vi "BRig_Host_dataRunState__entryDelete__delDataPlot.vi"(7 "input_idx":i32[](array[numeric]), 8 "input_col_dataPlot":u16, 9 "input_row_dataPlot":u16, 11 "input_dataPlot":u16[][](array[numeric])) -> (0 "output_arrTrials":bool, 3 "output_dataPlot":u16[][](array[numeric]), 4 "output_arrTrials_length":i32, 5 "output_idx":i32[](array[numeric]), 6 "output_arrTrials":i32[](array[numeric]))   [LabVIEW 2014]
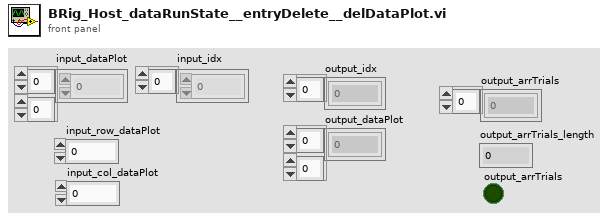
[diagram p1: front panel]
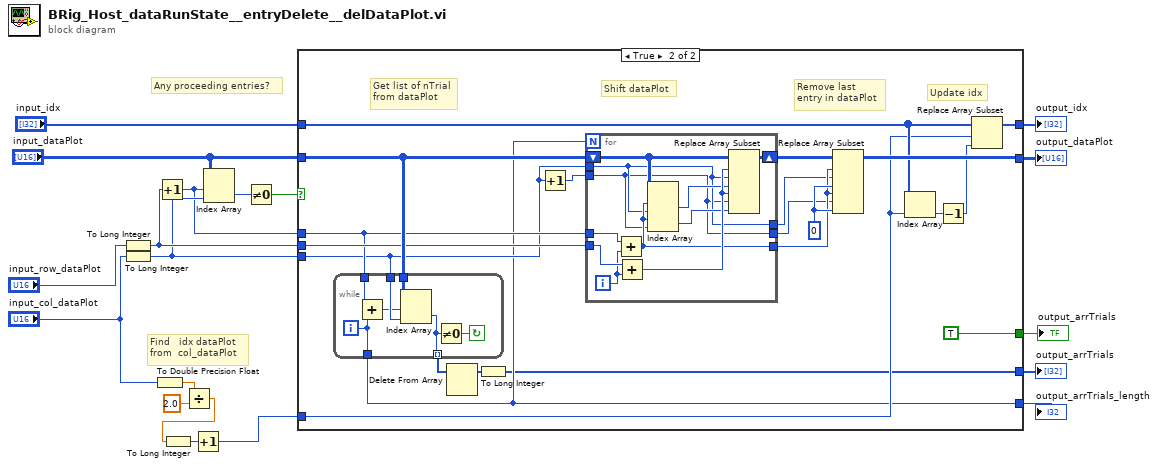
[diagram p0: block diagram]
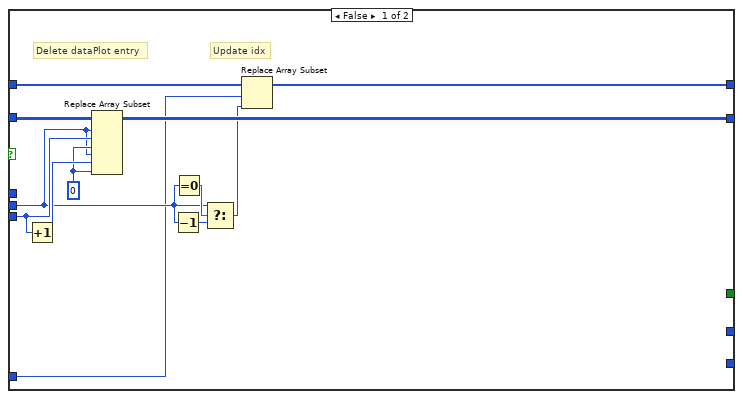
[diagram p2: hidden frame]
diagram:
  # "Find   idx dataPlot\nfrom  col_dataPlot"
  # "Any proceeding entries?"
  n1 = To Long Integer(number="input_row_dataPlot") -> (32bit integer=w14:i32)
  n2 = To Long Integer(number="input_col_dataPlot") -> (32bit integer=w13:i32)
  n3 = To Double Precision Float(number="input_col_dataPlot") -> (double precision float=w11:dbl)
  n4 = Increment(x=w14) -> (x+1=w12:i32)
  n5 = Divide(x=w11, y=2.0) -> (x/y=w9:dbl)
  n6 = To Long Integer(number=w9) -> (32bit integer=w8:i32)
  n7 = Increment(x=w8) -> (x+1=w6:i32)
  n8 = Index Array(array="input_dataPlot", index (row)=w12, index (col)=w13) -> (element=w18:u16)
  n9 = Not Equal To 0?(x=w18) -> (x != 0?=w17:bool)
  n10 = case shown="True" w17 {
    tunnel: "input_dataPlot" -> [w31 w51]
    tunnel: "input_idx" -> [w26 w39]
    tunnel: w14 -> [w22 w50]
    tunnel: w13 -> [w27 w48]
    tunnel: [w28 w41] -> w4
    tunnel: [w25 w40] -> w5
    tunnel: w12 -> [_ w49]
    tunnel: w6 -> [w20 w36]
    tunnel: [_ w32] -> w3
    tunnel: [_ w35] -> w2
    tunnel: [_ TRUE] -> w1
    frame False {
      w29 = u16 0 ("new element/subarray")
      # "Update idx"
      # "Delete dataPlot entry"
      n11 = Increment(x=w27) -> (x+1=w30:i32)
      n12 = Replace Array Subset(array=w31, new element #1=w29, index (row) #1=w22, index (col) #1=w27, new element #2=w29, index (row) #2=w22, index (col) #2=w30) -> (w28:u16[][])
      n13 = Decrement(x=w22) -> (x-1=w23:i32)
      n14 = Equal To 0?(x=w22) -> (x = 0?=w24:bool)
      n15 = Select(t=w22, s=w24, f=w23) -> (s? t:f=w21:i32)
      n16 = Replace Array Subset(array=w26, new element=w21, index=w20) -> (w25:i32[])
    }
    frame True {
      w46 = u16 0 ("new element/subarray")
      # "Update idx"
      # "Remove last\nentry in dataPlot"
      # "Shift dataPlot"
      # "Get list of nTrial\nfrom dataPlot"
      n17 = while {
        tunnel: w51 -> [w70]
        tunnel: w49 -> [w67]
        tunnel: w48 -> [w69]
        tunnel: [w65] -> w52 mode=indexing
        tunnel: [w64] -> w35
        i -> [w64]
        stop <- w66 continue-if-true
        n18 = Add(x=w67, y=w64) -> (x+y=w68:i32)
        n19 = Index Array(array=w70, index (row)=w68, index (col)=w69) -> (element=w65:u16)
        n20 = Not Equal To 0?(x=w65) -> (x != 0?=w66:bool)
      }
      n21 = Delete From Array(array=w52) -> (array with subset deleted=w33:u16[])  [unwired: 2 in, 1 out]
      n22 = To Long Integer(number=w33) -> (32bit integer=w32:i32[])
      n23 = Increment(x=w48) -> (x+1=w47:i32)
      n24 = for {
        N: w35 -> [_]
        shift-right: [w63] -> w45
        shift-left: w51 -> [w62]
        tunnel: w50 -> [w61]
        tunnel: w49 -> [w59]
        tunnel: w48 -> [w54]
        tunnel: w47 -> [w53]
        tunnel: [w55] -> w44
        tunnel: [w54] -> w43
        tunnel: [w53] -> w42
        i -> [w60]
        n25 = Add(x=w59, y=w60) -> (x+y=w55:i32)
        n26 = Add(x=w61, y=w60) -> (x+y=w58:i32)
        n27 = Index Array(array=w62, index (row) #1=w55, index (col) #1=w54, index (row) #2=w55, index (col) #2=w53) -> (element #1=w57:u16, element #2=w56:u16)
        n28 = Replace Array Subset(array=w62, new element #1=w57, index (row) #1=w58, index (col) #1=w54, new element #2=w56, index (row) #2=w58, index (col) #2=w53) -> (w63:u16[][])
      }
      n29 = Replace Array Subset(array=w45, new element #1=w46, index (row) #1=w44, index (col) #1=w43, new element #2=w46, index (row) #2=w44, index (col) #2=w42) -> (w41:u16[][])
      n30 = Index Array(array=w39, index=w36) -> (element=w38:i32)
      n31 = Decrement(x=w38) -> (x-1=w37:i32)
      n32 = Replace Array Subset(array=w39, new element=w37, index=w36) -> (w40:i32[])
    }
  }
  "output_idx" <- w5
  "output_dataPlot" <- w4
  "output_arrTrials" <- w3
  "output_arrTrials_length" <- w2
  "output_arrTrials" <- w1
